vi "顺序循环.vi"() -> ()   [LabVIEW 2017]
panel:
  out "x-y":u32
  out "布尔":bool
  in  "字符串":string
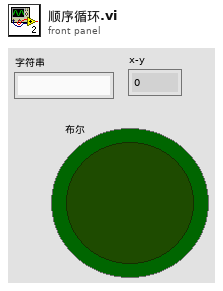
[diagram p1: front panel]
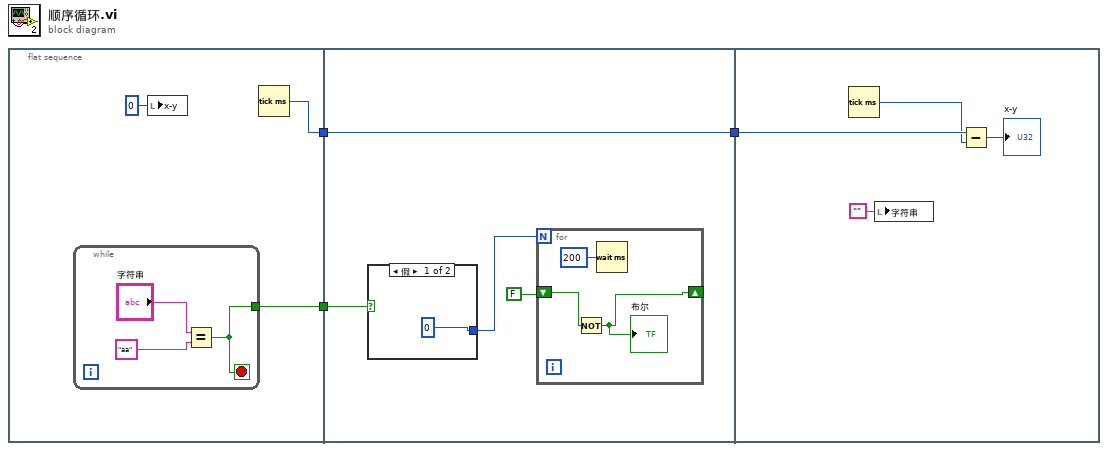
[diagram p0: block diagram]
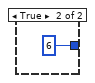
[diagram p2: hidden frame]
diagram:
  n1 = flat-sequence {
    tunnel: [w6] -> w2
    tunnel: [w4] -> w1
    tunnel: [w13] -> w3
    tunnel: w2 -> [w13]
    tunnel: w1 -> [w12]
    tunnel: w3 -> [w22]
    frame #0 {
      n2 = while {
        tunnel: [w7] -> w4
        stop <- w7 stop-if-true
        n3 = Equal?(x="字符串", y="aa") -> (x = y?=w7:bool)
      }
      n4 = local write "x-y"(u32 0 ("x-y")) -> ()
      n5 = Tick Count (ms)() -> (millisecond timer value=w6:u32)
    }
    frame #1 {
      n6 = case shown="假" w12 {
        tunnel: [0 6] -> w11
        frame False {
        }
        frame True {
        }
      }
      n7 = for {
        N: w11 -> [_]
        shift-right: [w14] -> _
        shift-left: FALSE -> [w15]
        n8 = Not(x=w15) -> (.not. x?=w14:bool)
        "布尔" <- w14
        n9 = Wait (ms)(milliseconds to wait=u32 200 ("等待时间（毫秒）")) -> ()  [unwired: 1 out]
      }
    }
    frame #2 {
      n10 = Tick Count (ms)() -> (millisecond timer value=w21:u32)
      n11 = local write "字符串"("" ("字符串")) -> ()
      n12 = Subtract(x=w22, y=w21) -> (x-y=→"x-y":u32)
    }
  }
